vi "RecordEvent.vi"(8 "error in (no error)":errorcluster, 9 "Event Description":string, 10 "Event Name":string, 11 "EventRecorder in":refnum<class "EventRecorder.lvclass">) -> (0 "error out":errorcluster, 3 "EventRecorder out":refnum<class "EventRecorder.lvclass">)   [LabVIEW 2019, in "EventRecorder.lvlib" / "EventRecorder.lvclass"]
uses:
  EventRecorder.lvclass
  EventRecorder.lvclass/EventRecorder.ctl
  <vilib>/NI/Event Logger Library/EventLog/EventLog.lvclass
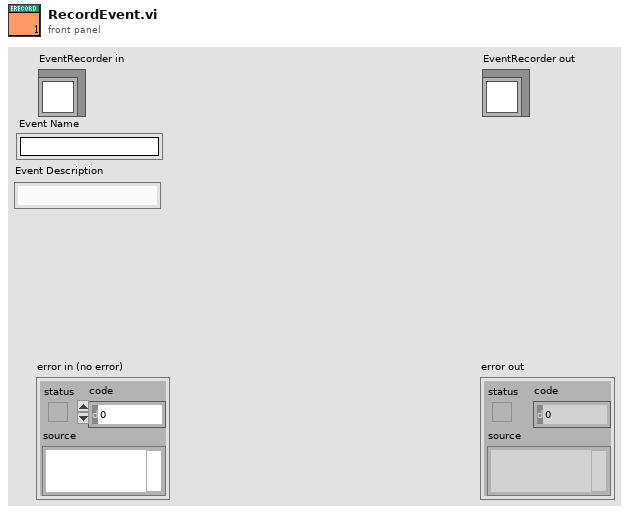
[diagram p1: front panel]
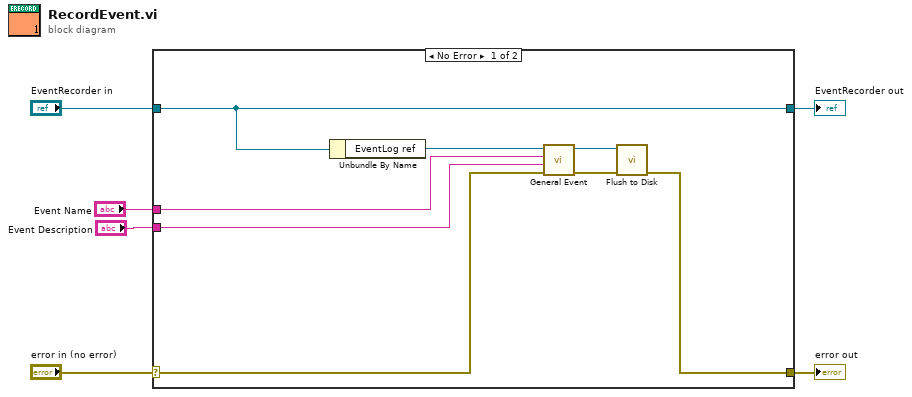
[diagram p0: block diagram]
diagram:
  n1 = case shown="No Error" "error in (no error)" {
    selector: "error in (no error)" -> [w12 w16]
    tunnel: [w7 w16] -> w5
    tunnel: [w14 w15] -> w3
    tunnel: "EventRecorder in" -> [w14 w15]
    tunnel: "Event Description" -> [w11 _]
    tunnel: "Event Name" -> [w10 _]
    frame No Error {
      n2 = Unbundle By Name(w14) -> ("EventLog ref"=w13:refnum<class "EventLog.lvclass">)
      n3 = call <vilib>:"General Event.vi"("error in (no error)"=w12, "Event Description"=w11, "Event Name"=w10, "EventLog ref"=w13) -> ("error out"=w8:errorcluster, "EventLog ref"=w9:refnum<class "EventLog.lvclass">)  [unwired: 6 in]
      n4 = call <vilib>:"Flush to Disk.vi"("error in (no error)"=w8, "EventLog ref"=w9) -> ("error out"=w7:errorcluster)  [unwired: 8 in, 1 out]
    }
    frame Error {
    }
  }
  "error out" <- w5
  "EventRecorder out" <- w3
